vi "BNC555.PC Write PSDB.vi"(0 "i ref in":refnum<vi>, 5 "error IO":errorcluster) -> (14 "i ref out":refnum<vi>, 19 "error out":errorcluster)   [LabVIEW 2014, in "BNC555.lvlib"]
doc: "This is the proc case which writes data to the PHELIX shot data base."
uses:
  BNC555.lvlib
  CSPhelix/PH_PSDBWriter/PH_PSDBWriter.Boolean dataset.ctl
  CSPhelix/PH_PSDBWriter/PH_PSDBWriter.Numeric dataset.ctl
  CSPhelix/PH_PSDBWriter/PH_PSDBWriter.String dataset.ctl
  CSPhelix/PH_PSDBWriter/PH_PSDBWriter.lvlib
panel:
  in  "System.Sys Trig Mode":enum16{"Disabled", "Triggered", "Gated"}(ring)
  in  "System.Sys Mode":T1(ring)
  in  "Chan Mode":T2(ring)
  in  "Chan Gate Pol":enum16{"Normal", "Complement", "Inverted"}(ring)
  in  "Chan Pol Out":enum16{"Normal", "Complement", "Inverted"}(ring)
  in  "Chan Level Out":enum16{"TTL", "Adjustable", "35 Volt"}(ring)
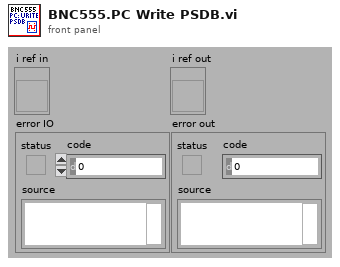
[diagram p1: front panel]
types:
  T1 = enum16{"Normal", "Single", "Burst", "Duty Cycle"}
  T2 = enum16{"Normal", "Single", "Burst", "Divide by N"}
  T3 = typedef "PH_PSDBWriter.lvlib/PH_PSDBWriter.String dataset.ctl" = cluster{"name":string, "data":string, "unit":string}
  T4 = typedef "PH_PSDBWriter.lvlib/PH_PSDBWriter.Numeric dataset.ctl" = cluster{"name":string, "data":dbl, "unit":string}
  T5 = typedef "PH_PSDBWriter.lvlib/PH_PSDBWriter.Boolean dataset.ctl" = cluster{"name":string, "data":bool, "unit":string}
  T6 = typedef "BNC555.lvlib/BNC555.i attribute.ctl" = cluster{"Information":cluster{"VISA resource name":refnum<visa-resource-name>, "Baud Rate (1:9600)":u16}, "Channel Array":T7[], "System":T8, "GUI Refs":cluster{"Delete":refnum<vi>, "Information":refnum<vi>, "System":refnum<vi>, "Channel Array":refnum<vi>, "Device Error":refnum<vi>, "Instr Driver Revision":refnum<vi>, "Instr Firmware Revision":refnum<vi>, "Instr Option":refnum<vi>, "Self-Test Response":refnum<vi>}, "Service IDs Channelinfo":i32[], "Service ID T0 Mode":i32}
  T7 = typedef "BNC555 - Driver np.lvlib/BNC555 All Chan Parameters.ctl" = cluster{"Chan #":i32, "Chan State":bool, "Chan Delay":dbl, "Chan Width":dbl, "Chan Mode":enum16{"Normal", "Single", "Burst", "Divide by N"}, "Chan Burst #":u32, "Chan Divide #":u32, "Chan Pol Out":enum16{"Normal", "Complement", "Inverted"}, "Chan Level Out":enum16{"TTL", "Adjustable", "35 Volt"}, "Chan Lev Adjust":dbl, "Chan Gate Pol":enum16{"Normal", "Complement", "Inverted"}, "Chan Gate State":bool}
  T8 = typedef "BNC555 - Driver np.lvlib/BNC555 All Sys Parameters.ctl" = cluster{"Sys Period":dbl, "Sys Oscillator":bool, "Sys Mode":enum16{"Normal", "Single", "Burst", "Duty Cycle"}, "Sys Burst #":u32, "Sys DC On":u32, "Sys DC Off":u32, "Sys Trig Mode":enum16{"Disabled", "Triggered", "Gated"}, "Sys Trig Lev":dbl, "Sys Gate State":bool, "Sys Trig Edge":bool, "Sys State":bool}
  T9 = typedef "PH_PSDBWriter.lvlib/PH_PSDBWriter.PSDB Dataset.ctl" = cluster{"Version":i32, "2D data Input":T10[], "Boolean Input":T5[], "Image Input":T12[], "Numeric Input":T4[], "String Input":T3[]}
  T10 = typedef "PH_PSDBWriter.lvlib/PH_PSDBWriter.2D dataset.ctl" = cluster{"name":string, "data":dbl[][], "axis description":T11}
  T11 = typedef "PSDB.lvlib/PSDB_AxisDescription.ctl" = cluster{"x axis label":string, "y axis label":string, "x axis unit":string, "y axis unit":string}
  T12 = typedef "PH_PSDBWriter.lvlib/PH_PSDBWriter.Image dataset.ctl" = cluster{"name":string, "data":T13, "unit":string}
  T13 = typedef "IMAQ Image.ctl" = refnum<image>
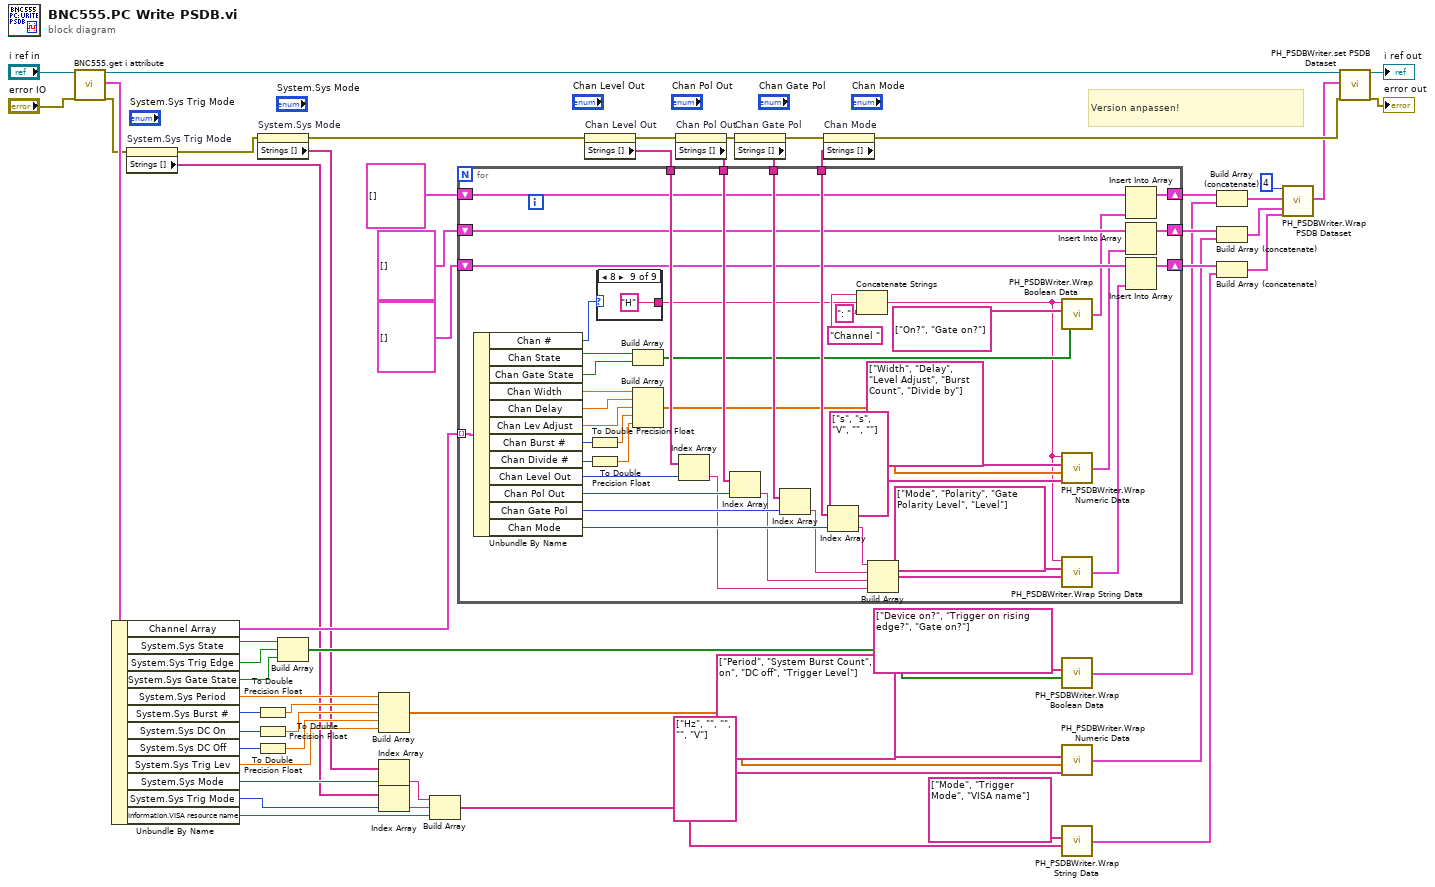
[diagram p0: block diagram]
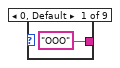
[diagram p2: hidden frame]
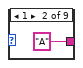
[diagram p3: hidden frame]
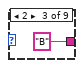
[diagram p4: hidden frame]
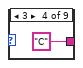
[diagram p5: hidden frame]
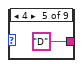
[diagram p6: hidden frame]
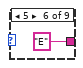
[diagram p7: hidden frame]
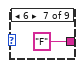
[diagram p8: hidden frame]
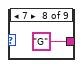
[diagram p9: hidden frame]
diagram:
  # "Version anpassen!"
  n1 = call "BNC555.get i attribute.vi"("i ref in"="i ref in", "error in (no error)"="error IO") -> ("i ref out"=w55:refnum<vi>, "i attribute"=w53:T6, "error out"=w4:errorcluster)  [unwired: 15 in]
  n2 = Unbundle By Name(w53) -> ("Channel Array"=w54:T7[], "System.Sys State"=w42:bool, "System.Sys Trig Edge"=w43:bool, "System.Sys Gate State"=w44:bool, "System.Sys Period"=w39:dbl, "System.Sys Burst #"=w38:u32, "System.Sys DC On"=w37:u32, "System.Sys DC Off"=w36:u32, "System.Sys Trig Lev"=w33:dbl, "System.Sys Mode"=w28:T1, "System.Sys Trig Mode"=w27:enum16{"Disabled", "Triggered", "Gated"}, "Information.VISA resource name"=w24:refnum<visa-resource-name>)
  n3 = property on="System.Sys Trig Mode" class="Enum (strict)"(error in=w4) -> (error out=w3:errorcluster, "Strings []"=w1:string[])  [unwired: 1 in, 1 out]
  n4 = property on="System.Sys Mode" class="Enum (strict)"(error in=w3) -> (error out=w2:errorcluster, "Strings []"=w5:string[])  [unwired: 1 in, 1 out]
  n5 = To Double Precision Float(number=w38) -> (double precision float=w35:dbl)
  n6 = To Double Precision Float(number=w37) -> (double precision float=w34:dbl)
  n7 = To Double Precision Float(number=w36) -> (double precision float=w40:dbl)
  n8 = Build Array(w42, w43, w44) -> (w11:bool[])
  n9 = Build Array(w39, w35, w34, w40, w33) -> (w13:dbl[])
  n10 = Index Array(array=w5, index=w28) -> (element=w26:string)
  n11 = Index Array(array=w1, index=w27) -> (element=w25:string)
  n12 = Build Array(w26, w25, w24) -> (w6:string[])
  n13 = property on="Chan Level Out" class="Enum (strict)"(error in=w2) -> (error out=w48:errorcluster, "Strings []"=w49:string[])  [unwired: 1 in, 1 out]
  n14 = property on="Chan Pol Out" class="Enum (strict)"(error in=w48) -> (error out=w47:errorcluster, "Strings []"=w50:string[])  [unwired: 1 in, 1 out]
  n15 = property on="Chan Gate Pol" class="Enum (strict)"(error in=w47) -> (error out=w46:errorcluster, "Strings []"=w51:string[])  [unwired: 1 in, 1 out]
  n16 = property on="Chan Mode" class="Enum (strict)"(error in=w46) -> (error out=w22:errorcluster, "Strings []"=w52:string[])  [unwired: 1 in, 1 out]
  n17 = for {
    tunnel: w54 -> [w100] mode=indexing
    tunnel: w52 -> [w94]
    tunnel: w51 -> [w93]
    tunnel: w50 -> [w92]
    tunnel: w49 -> [w91]
    shift-right: [w74] -> w41
    shift-left: T5[] [] -> [w73]
    shift-right: [w72] -> w32
    shift-left: T4[] [] -> [w71]
    shift-right: [w70] -> w29
    shift-left: T3[] [] -> [w69]
    n18 = Unbundle By Name(w100) -> ("Chan #"=w99:i32, "Chan State"=w79:bool, "Chan Gate State"=w78:bool, "Chan Width"=w84:dbl, "Chan Delay"=w83:dbl, "Chan Lev Adjust"=w82:dbl, "Chan Burst #"=w86:u32, "Chan Divide #"=w85:u32, "Chan Level Out"=w98:enum16{"TTL", "Adjustable", "35 Volt"}, "Chan Pol Out"=w97:enum16{"Normal", "Complement", "Inverted"}, "Chan Gate Pol"=w96:enum16{"Normal", "Complement", "Inverted"}, "Chan Mode"=w95:T2)
    n19 = To Double Precision Float(number=w86) -> (double precision float=w81:dbl)
    n20 = To Double Precision Float(number=w85) -> (double precision float=w80:dbl)
    n21 = case shown="8" w99 {
      tunnel: ["OOO" "A" "B" "C" "D" "E" "F" "G" "H"] -> w76
      frame 0, Default {
      }
      frame 1 {
      }
      frame 2 {
      }
      frame 3 {
      }
      frame 4 {
      }
      frame 5 {
      }
      frame 6 {
      }
      frame 7 {
      }
      frame 8 {
      }
    }
    n22 = Build Array(w79, w78) -> (w67:bool[])
    n23 = Build Array(w84, w83, w82, w81, w80) -> (w65:dbl[])
    n24 = Index Array(array=w91, index=w98) -> (element=w90:string)
    n25 = Index Array(array=w92, index=w97) -> (element=w89:string)
    n26 = Index Array(array=w93, index=w96) -> (element=w88:string)
    n27 = Index Array(array=w94, index=w95) -> (element=w87:string)
    n28 = Concatenate Strings("Channel ", w76, ": " ("string")) -> (w60:string)
    n29 = Build Array(w87, w88, w89, w90) -> (w58:string[])
    n30 = call "PH_PSDBWriter.Wrap Boolean Data.vi"("Data Array"=w67, "Name Array"=string[] ["On?", "Gate on?"], "Name Prefix"=w60) -> ("PSDB Boolean Data Array"=w66:T5[])  [unwired: 1 in]
    n31 = call "PH_PSDBWriter.Wrap Numeric Data.vi"("Unit Array"=string[] ["s", "s", "V", "", ""], "Data Array"=w65, "Name Array"=string[] ["Width", "Delay", "Level Adjust", "Burst Count", "Divide by"], "Name Prefix"=w60) -> ("PSDB Numeric Data Array"=w62:T4[])
    n32 = call "PH_PSDBWriter.Wrap String Data.vi"("Data Array"=w58, "Name Array"=string[] ["Mode", "Polarity", "Gate Polarity Level", "Level"], "Name Prefix"=w60) -> ("PSDB String Data Array"=w61:T3[])  [unwired: 1 in]
    n33 = Insert Into Array(array=w73, new element=w66) -> (w74:T5[])  [unwired: 1 in]
    n34 = Insert Into Array(array=w71, new element=w62) -> (w72:T4[])  [unwired: 1 in]
    n35 = Insert Into Array(array=w69, new element=w61) -> (w70:T3[])  [unwired: 1 in]
  }
  n36 = call "PH_PSDBWriter.Wrap Boolean Data.vi"("Data Array"=w11, "Name Array"=string[] ["Device on?", "Trigger on rising edge?", "Gate on?"]) -> ("PSDB Boolean Data Array"=w9:T5[])  [unwired: 2 in]
  n37 = call "PH_PSDBWriter.Wrap Numeric Data.vi"("Unit Array"=string[] ["Hz", "", "", "", "V"], "Data Array"=w13, "Name Array"=string[] ["Period", "System Burst Count", "DC on", "DC off", "Trigger Level"]) -> ("PSDB Numeric Data Array"=w12:T4[])  [unwired: 1 in]
  n38 = call "PH_PSDBWriter.Wrap String Data.vi"("Data Array"=w6, "Name Array"=string[] ["Mode", "Trigger Mode", "VISA name"]) -> ("PSDB String Data Array"=w8:T3[])  [unwired: 2 in]
  n39 = Build Array (concatenate)(w41, w9) -> (w18:T5[])
  n40 = Build Array (concatenate)(w32, w12) -> (w17:T4[])
  n41 = Build Array (concatenate)(w29, w8) -> (w16:T3[])
  n42 = call "PH_PSDBWriter.Wrap PSDB Dataset.vi"("Version"=4, "Boolean Input"=w18, "Numeric Input"=w17, "String Input"=w16) -> ("PSDB Dataset"=w19:T9)  [unwired: 15 in]
  n43 = call "PH_PSDBWriter.set PSDB Dataset.vi"("VI in"=w55, "PSDB Dataset"=w19, "error in (no error)"=w22) -> ("VI out"=→"i ref out":refnum<vi>, "error out"=→"error out":errorcluster)  [unwired: 15 in]
